vi "Pockels-Generate ref frame seq insertion indexes.vi"(7 "Prevent small final chunks (T)":bool=TRUE, 9 "Nominal chunk length (points)":i32, 10 "Number of POI":i32=3, 11 "Number of points in the original pockels modulation sequence":i32) -> (1 "Insertion indexes":i32[](array[numeric]), 2 "Size of last chunk as % of nominal chunk size":dbl(slide) scale=0.0..100.0, 3 "Number of insertions":i32)   [LabVIEW 2020]
panel:
  out "Nominal chunk length (points) normalised to POI resolution":i32
  out "Nominal number of POI":i32
  out "Points per POI":i32=3
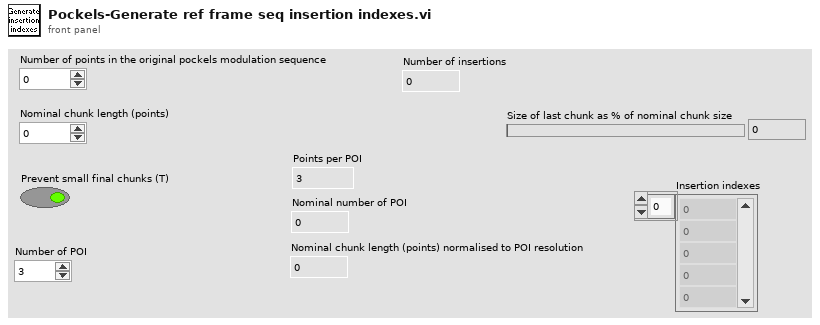
[diagram p1: front panel]
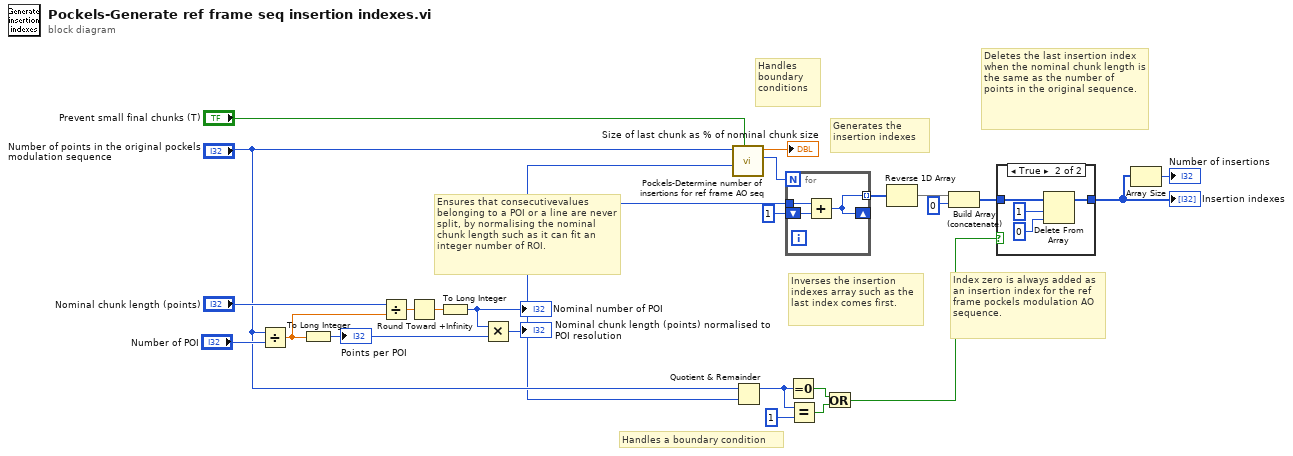
[diagram p0: block diagram]
diagram:
  # "Ensures that consecutivevalues belonging to a POI or a line are never split, by normalising the nominal chunk length such as it can fit an integer number of ROI."
  # "Handles a boundary condition"
  # "Deletes the last insertion index when the nominal chunk length is the same as the number of points in the original sequence."
  # "Index zero is always added as an insertion index for the ref frame pockels modulation AO sequence."
  # "Handles boundary conditions"
  # "Inverses the insertion indexes array such as the last index comes first."
  # "Generates the insertion indexes"
  n1 = Divide(x="Number of points in the original pockels modulation sequence", y="Number of POI") -> (x/y=w1:dbl)
  n2 = To Long Integer(number=w1) -> (32bit integer=w15:i32)
  "Points per POI" <- w15
  n3 = Divide(x="Nominal chunk length (points)", y=w1) -> (x/y=w14:dbl)
  n4 = Round Toward +Infinity(x=w14) -> (ceil(x): smallest int >= x=w13:dbl)
  n5 = To Long Integer(number=w13) -> (32bit integer=w12:i32)
  "Nominal number of POI" <- w12
  n6 = Multiply(x=w12, y=w15) -> (x*y=w7:i32)
  "Nominal chunk length (points) normalised to POI resolution" <- w7
  n7 = call "Pockels-Determine number of insertions for ref frame AO seq.vi"("Prevent small final chunks (T)"="Prevent small final chunks (T)", "Nominal chunk length (points)"=w7, "Number of points in the original pockels modulation sequence"="Number of points in the original pockels modulation sequence") -> ("Number of insertions"=w23:i32, "Size of last chunk as % of nominal chunk size"=→"Size of last chunk as % of nominal chunk size":dbl)  [unwired: 7 in]
  n8 = Quotient & Remainder(x="Number of points in the original pockels modulation sequence", y=w7) -> (x-y*floor(x/y)=w6:i32)  [unwired: 1 out]
  n9 = for {
    N: w23 -> [_]
    tunnel: w7 -> [w27]
    shift-right: [w25] -> _
    shift-left: 1 -> [w26]
    tunnel: [w25] -> w19 mode=indexing
    n10 = Add(x=w27, y=w26) -> (x+y=w25:i32)
  }
  n11 = Equal To 0?(x=w6) -> (x = 0?=w3:bool)
  n12 = Equal?(x=w6, y=1) -> (x = y?=w4:bool)
  n13 = Or(x=w3, y=w4) -> (x .or. y?=w2:bool)
  n14 = Reverse 1D Array(array=w19) -> (reversed array=w20:i32[])
  n15 = Build Array (concatenate)(w20, 0) -> (w10:i32[])
  n16 = case shown="True" w2 {
    tunnel: w10 -> [w28 w32]
    tunnel: [w28 w31] -> w9
    frame False {
    }
    frame True {
      n17 = Delete From Array(array=w32, length=1, index=0) -> (array with subset deleted=w31:i32[])  [unwired: 1 out]
    }
  }
  "Insertion indexes" <- w9
  n18 = Array Size(array=w9) -> (size(s)=→"Number of insertions":i32)
